vi "Position Numeric Done Key.vi"(8 "error in (no error)":errorcluster, 10 "0 Key":refnum<vi>, 11 "Done Key":refnum<vi>) -> (0 "error out":errorcluster)   [LabVIEW 2014]
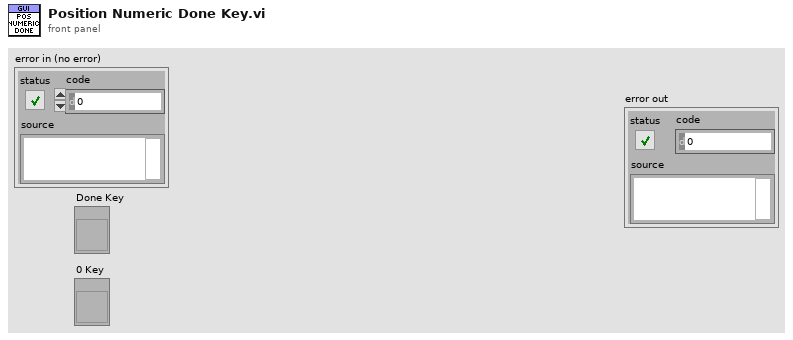
[diagram p1: front panel]
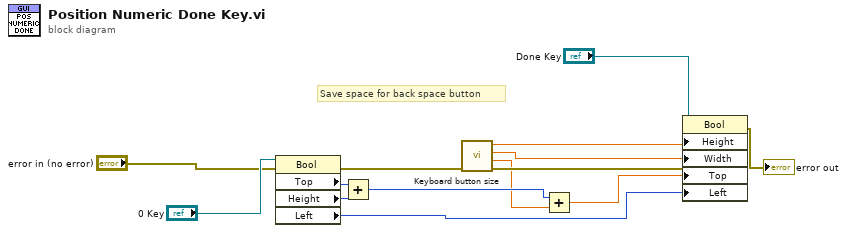
[diagram p0: block diagram]
diagram:
  # "Save space for back space button"
  n1 = property class="Bool"(reference="0 Key", error in="error in (no error)") -> (error out=w11:errorcluster, "Top"=w13:i32, "Height"=w12:u32, "Left"=w1:i32)  [unwired: 1 out]
  n2 = Add(x=w13, y=w12) -> (x+y=w7:u32)
  n3 = call "Keyboard button size.vi"("error in (no error)"=w11) -> ("error out"=w9:errorcluster, "Key Spacing"=w6:dbl, "Key Width"=w5:dbl, "Key Height"=w4:dbl)  [unwired: 7 in]
  n4 = Add(x=w7, y=w6) -> (x+y=w2:dbl)
  n5 = property class="Bool"(reference="Done Key", error in=w9, "Height"=w4, "Width"=w5, "Top"=w2, "Left"=w1) -> (error out=→"error out":errorcluster)  [unwired: 1 out]
